vi "5_4.vi"() -> ()   [LabVIEW 2018]
uses:
  <vilib>/gmath/NI_Gmath.lvlib
panel:
  out "观测次数m":i32
  out "理论最佳误码率":dbl
  in  "观测时刻（0-1）":dbl[](array[numeric])
  out "噪声标准差":dbl
  out "设计误码率":ext
  out "理论最优门限":dbl
  out "先验概率P(H1)":dbl
  in  "先验概率P(H0)":dbl=0.5
  in  "噪声方差":dbl=0.5
  in  "样本数":u64=1000000
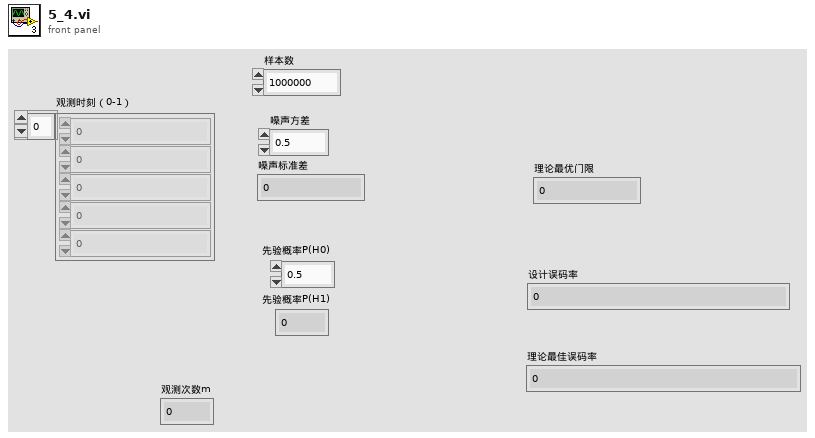
[diagram p1: front panel]
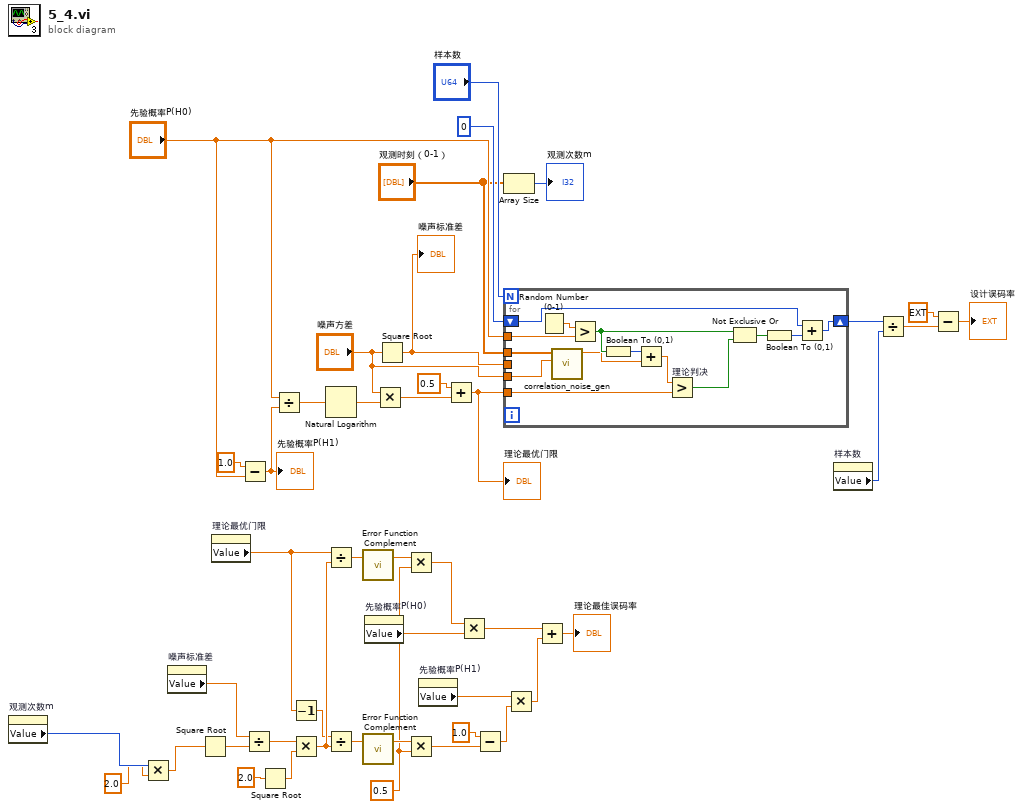
[diagram p0: block diagram]
diagram:
  w19 = 0.5 ("y")
  n1 = property on="观测次数m" class="DigNum (严格)"() -> ("Value"=w3:i32)  [unwired: 2 in, 2 out]
  n2 = Multiply(x=w3, y=2.0 ("x")) -> (x*y=w1:dbl)
  n3 = property on="噪声标准差" class="DigNum (严格)"() -> ("Value"=w8:dbl)  [unwired: 2 in, 2 out]
  n4 = Square Root(x=w1) -> (sqrt(x)=w11:dbl)
  n5 = property on="理论最优门限" class="DigNum (严格)"() -> ("Value"=w9:dbl)  [unwired: 2 in, 2 out]
  n6 = Subtract(x=1.0, y="先验概率P(H0)") -> (x-y=w37:dbl)
  "先验概率P(H1)" <- w37
  n7 = Divide(x=w8, y=w11) -> (x/y=w10:dbl)
  n8 = Square Root(x=2.0) -> (sqrt(x)=w26:dbl)
  n9 = Divide(x="先验概率P(H0)", y=w37) -> (x/y=w42:dbl)
  n10 = Decrement(x=w9) -> (x-1=w24:dbl)
  n11 = Multiply(x=w10, y=w26) -> (x*y=w25:dbl)
  n12 = Natural Logarithm(1:w42) -> (0:w41:dbl)
  n13 = Divide(x=w9, y=w25) -> (x/y=w23:dbl)
  n14 = Divide(x=w24, y=w25) -> (x/y=w22:dbl)
  n15 = call <vilib>:"Error Function Complement.vi"("x"=w23) -> ("1 - erf(x)"=w20:dbl)  [unwired: 2 in]
  n16 = call <vilib>:"Error Function Complement.vi"("x"=w22) -> ("1 - erf(x)"=w21:dbl)  [unwired: 2 in]
  n17 = property on="先验概率P(H0)" class="DigNum (严格)"() -> ("Value"=w5:dbl)  [unwired: 2 in, 2 out]
  n18 = Multiply(x="噪声方差", y=w41) -> (x*y=w40:dbl)
  n19 = Square Root(x="噪声方差") -> (sqrt(x)=w31:dbl)
  "噪声标准差" <- w31
  n20 = Multiply(x=w20, y=w19) -> (x*y=w15:dbl)
  n21 = Multiply(x=w21, y=w19) -> (x*y=w18:dbl)
  n22 = property on="先验概率P(H1)" class="DigNum (严格)"() -> ("Value"=w4:dbl)  [unwired: 2 in, 2 out]
  n23 = Add(x=0.5, y=w40) -> (x+y=w35:dbl)
  "理论最优门限" <- w35
  n24 = Multiply(x=w15, y=w5) -> (x*y=w12:dbl)
  n25 = Subtract(x=1.0, y=w18) -> (x-y=w14:dbl)
  n26 = Array Size(array="观测时刻（0-1）") -> (size(s)=→"观测次数m":i32)
  n27 = for {
    N: "样本数" -> [_]
    tunnel: "先验概率P(H0)" -> [w57]
    tunnel: w35 -> [w56]
    shift-right: [w54] -> w30
    shift-left: u64 0 ("元素") -> [w52]
    tunnel: w31 -> [_]
    tunnel: "噪声方差" -> [w48]
    tunnel: "观测时刻（0-1）" -> [w47]
    n28 = Random Number (0-1)() -> (number: 0 to 1=w58:dbl)
    n29 = call "correlation_noise_gen.vi"("噪声方差"=w48, "观测时刻（0-1）"=w47) -> ("平均观测噪声"=w46:dbl)  [unwired: 9 in]
    n30 = Greater?(x=w58, y=w57) -> (0:w49:bool)
    n31 = Boolean To (0,1)(Boolean=w49) -> (0, 1=w51:i16)
    n32 = Add(x=w51, y=w46) -> (x+y=w45:dbl)
    n33 = Greater? "理论判决"(x=w45, y=w56) -> (0:w55:bool)
    n34 = Not Exclusive Or(1:w55, 2:w49) -> (0:w50:bool)
    n35 = Boolean To (0,1)(Boolean=w50) -> (0, 1=w53:i16)
    n36 = Add(x=w52, y=w53) -> (x+y=w54:u64)
  }
  n37 = Multiply(x=w4, y=w14) -> (x*y=w13:dbl)
  n38 = Add(x=w12, y=w13) -> (x+y=→"理论最佳误码率":dbl)
  n39 = property on="样本数" class="DigNum (严格)"() -> ("Value"=w29:u64)  [unwired: 2 in, 2 out]
  n40 = Divide(x=w30, y=w29) -> (x/y=w34:dbl)
  n41 = Subtract(x=ext 1.0, y=w34) -> (x-y=→"设计误码率":ext)
